vi "deinitialize.vi"(0 "HGF_ThreadTask":refnum<class "HGF_ThreadTask.lvclass">, 5 "error in (no error)":errorcluster) -> (19 "error out":errorcluster)   [LabVIEW 2014, in "HGF_BaseClasses.lvlib" / "HGF_ThreadTask.lvclass"]
doc: "This is a dynamic dispatch VI. It can be overwritten by childclasses to release allocated recources."
uses:
  HGF_ThreadTask.lvclass
  HGF_Factory/HGF_Factory.lvclass
  HGF_Base/HGF_Base.lvclass
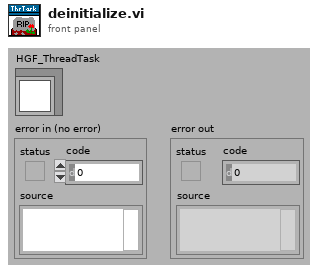
[diagram p1: front panel]
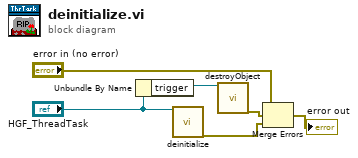
[diagram p0: block diagram]
diagram:
  n1 = Unbundle By Name("HGF_ThreadTask") -> ("trigger"=w5:refnum<class "HGF_Event.lvclass">)
  n2 = call-parent "deinitialize.vi"("HGF_Factory"="HGF_ThreadTask") -> ("error out"=w1:errorcluster)  [unwired: 1 in, 17 out]
  n3 = call "destroyObject.vi"("HGF_Factory"=w5) -> ("error out"=w2:errorcluster)  [unwired: 18 in]
  n4 = Merge Errors("error in (no error)", w2, w1) -> (→"error out":errorcluster)
